vi "Sequencer Main - Copy.vi"() -> ()   [LabVIEW 2018] (continued)
                                }
                                frame True {
                                # "if(Retest-OFF & Cnt=0)"
                                n1515 = Decrement(x=w2562) -> (x-1=w2561:i32)
                                n1516 = global write "Global Variable.vi" "Retest Cnt"(w2561) -> ()
                                }
                                }
                                n1517 = global write "Global Variable.vi" "Retest ON"(TRUE ("Retest ON")) -> ()
                                }
                                }
                                }
                                frame True {
                                }
                              }
                            }
                          }
                        }
                        frame 42 {
                          # "BlueTooht Case\nEsp32 Reset"
                          # "Test ADB Bluetooth"
                          n1518 = Unbundle By Name(w2603) -> ("Parameters"=w2594:string, "Step Description"=w2591:string, "Test Values.Upper Limit"=w2598:dbl, "Test Values.Lower Limit"=w2597:dbl)  [unwired: 1 out]
                          n1519 = in-place {
                            in-place-border: w2594 -> [w2673]
                            in-place-border: [w2669] -> w2593
                            in-place-border: [w2668] -> w2592
                            # "Str \"fase\" exist"
                            n1520 = To Lower Case(string=w2673) -> (all lower case string=w2674:string)
                            n1521 = Match Pattern(string=w2674, regular expression="false") -> (after substring=w2671:string, offset past match=w2670:i32)  [unwired: 1 in, 2 out]
                            n1522 = Greater Or Equal To 0?(x=w2670) -> (x >= 0?=w2668:bool)
                            n1523 = case shown="True" w2668 {
                              tunnel: w2671 -> [_ w2677]
                              tunnel: [string[] [] w2676] -> w2669
                              frame False {
                                (unwired) ""
                              }
                              frame True {
                                n1524 = while {
                                shift-right: [w2681] -> _
                                shift-left: w2677 -> [w2682]
                                tunnel: [w2678] -> w2676 mode=indexing
                                stop <- w2680 stop-if-true
                                # "Get Array of Sub Parametrs"
                                n1525 = Match Pattern(string=w2682, regular expression=":") -> (before substring=w2678:string, after substring=w2681:string, offset past match=w2679:i32)  [unwired: 1 in, 1 out]
                                n1526 = Less Than 0?(x=w2679) -> (x < 0?=w2680:bool)
                                }
                              }
                            }
                          }
                          n1527 = property on="Msg Str" class="Str"("Value"=w2591) -> ()  [unwired: 2 in, 2 out]
                          n1528 = global read "Global Variable.vi" "COM Port BLE"() -> (w2588:refnum<visa-resource-name>)
                          n1529 = invoke on="Serial CMD Mon" class="Str" method="Reinit To Default"() -> (error out=w2587:errorcluster)  [unwired: 3 in, 2 out]
                          n1530 = property on="Tab Control Msg" class="TabCtl (strict)"("Value"=T4."Serial" ("Tab Control Msg")) -> (error out=w2601:errorcluster)  [unwired: 2 in, 1 out]
                          n1531 = flat-sequence {
                            tunnel: w2601 -> [w2611]
                            tunnel: w2598 -> [_]
                            tunnel: w2597 -> [_]
                            tunnel: w2594 -> [w2610]
                            tunnel: [w2612] -> w2596
                            tunnel: ["Reset ESP_32"] -> w2595
                            tunnel: w2591 -> [w2609]
                            tunnel: [w2604] -> w2590
                            tunnel: [w2608] -> w2589
                            tunnel: w2588 -> [w2607]
                            tunnel: w2587 -> [_]
                            tunnel: [w2632] -> w2599
                            tunnel: [w2638] -> w2602
                            tunnel: w2596 -> [w2638]
                            tunnel: w2595 -> [w2632]
                            tunnel: w2593 -> [w2637]
                            tunnel: w2592 -> [w2635]
                            tunnel: w2590 -> [w2631]
                            tunnel: w2589 -> [w2630]
                            frame #0 {
                              # "Step TEST Description"
                              # "Step TEST Result"
                              n1532 = in-place {
                                in-place-border: w2610 -> [w2619]
                                in-place-border: w2611 -> [_]
                                in-place-border: w2609 -> [w2617]
                                in-place-border: [w2616] -> w2604
                                in-place-border: [w2617] -> w2608
                                in-place-border: w2607 -> [w2618]
                                in-place-border: [w2615] -> w2605
                                # "ADB BLE Name"
                                n1533 = while {
                                shift-right: [w2627] -> _
                                shift-left: w2619 -> [w2628]
                                tunnel: [w2624] -> w2620 mode=indexing
                                stop <- w2626 stop-if-true
                                # "Get Array of Parametrs"
                                n1534 = Match Pattern(string=w2628, regular expression=">") -> (before substring=w2624:string, after substring=w2627:string, offset past match=w2625:i32)  [unwired: 1 in, 1 out]
                                n1535 = Less Than 0?(x=w2625) -> (x < 0?=w2626:bool)
                                }
                                n1536 = call "ADB-LMS_Esp32_Rst.vi"("COM BLE Esp32"=w2618) -> ("Stat"=w2615:bool, "CMD Monitor"=w2616:string)  [unwired: 9 in]
                                n1537 = Index Array(array=w2620, index #1=0 ("index"), index #2=1 ("index"), index #3=2 ("index")) -> ()  [unwired: 3 out]
                              }
                              n1538 = local write "Serial CMD Mon"(w2604) -> ()
                              n1539 = case shown="True" w2605 {
                                tunnel: [enum16{"Idle", "PASS", "FALSE"}."FALSE" ("Step Test Result") enum16{"Idle", "PASS", "FALSE"}."PASS" ("Step Test Result")] -> w2612
                                frame False {
                                }
                                frame True {
                                }
                              }
                            }
                            frame #1 {
                              # "Str \"fase\" Present"
                              n1540 = in-place {
                                in-place-border: w2630 -> [w2641]
                                in-place-border: w2631 -> [w2640]
                                in-place-border: w2632 -> [w2639]
                                n1541 = call "Log Add Msg.vi"("Result"=w2639, "Communication"=w2640, "Description"=w2641) -> ("Out Msg"=w2642:string)
                                n1542 = property on="LogMsg" class="Str"("Text.Scroll Position"=inf) -> ()  [unwired: 2 in, 2 out]
                                n1543 = invoke on="LogMsg" class="Str" method="Append String"("string"=w2642) -> ()  [unwired: 3 in, 4 out]
                              }
                              n1544 = in-place {
                                in-place-border: w2637 -> [w2667]
                                in-place-border: [w2661] -> w2634
                                in-place-border: [w2660] -> w2633
                                # "GoTo Test-nmb"
                                # "ReTest Cyckles"
                                n1545 = Index Array(array=w2667, index #1=0, index #2=1, index #3=2) -> (element #2=w2663:string, element #3=w2662:string)  [unwired: 1 out]
                                n1546 = Decimal String To Number(string=w2663) -> (number=w2661:i32)  [unwired: 2 in, 1 out]
                                n1547 = Decimal String To Number(string=w2662) -> (number=w2660:i32)  [unwired: 2 in, 1 out]
                              }
                              n1548 = local read "Debugging"() -> (w2636:bool)
                              n1549 = case shown="False" w2636 {
                                tunnel: w2635 -> [w2647 _]
                                tunnel: w2634 -> [w2645 _]
                                tunnel: w2633 -> [w2644 _]
                                frame False {
                                # "No Debug Mode"
                                n1550 = in-place {
                                in-place-border: [w2649] -> w2646
                                n1551 = global read "Global Variable.vi" "Retest Cnt"() -> (w2650:i16)
                                n1552 = Equal?(x=w2650, y=i16 0) -> (x = y?=w2649:bool)
                                }
                                n1553 = case shown="True" w2647 {
                                tunnel: w2646 -> [_ w2654]
                                tunnel: w2645 -> [_ w2652]
                                tunnel: w2644 -> [_ w2651]
                                frame False {
                                }
                                frame True {
                                # "String \"false\" Present"
                                n1554 = global write "Global Variable.vi" "Retest Step Nmb"(w2652) -> ()
                                n1555 = global write "Global Variable.vi" "Retest Nmb"(w2651) -> ()
                                n1556 = case shown="False" w2654 {
                                tunnel: w2651 -> [_ w2659]
                                frame False {
                                n1557 = global read "Global Variable.vi" "Retest Cnt"() -> (w2657:i16)
                                n1558 = Decrement(x=w2657) -> (x-1=w2656:i16)
                                n1559 = global write "Global Variable.vi" "Retest Cnt"(w2656) -> ()
                                n1560 = Wait (ms)(milliseconds to wait=u32 1000) -> ()  [unwired: 1 out]
                                }
                                frame True {
                                # "if(Retest-OFF & Cnt=0)"
                                n1561 = Decrement(x=w2659) -> (x-1=w2658:i32)
                                n1562 = global write "Global Variable.vi" "Retest Cnt"(w2658) -> ()
                                }
                                }
                                n1563 = global write "Global Variable.vi" "Retest ON"(TRUE ("Retest ON")) -> ()
                                }
                                }
                                }
                                frame True {
                                }
                              }
                            }
                          }
                        }
                        frame 43 {
                          w2700 = "------------------------" ("string")
                          w2699 = "\r\n"
                          # "Step TEST Result"
                          # "Step Result Msg"
                          # "Str with \"false\" goto parameters"
                          # "Str \"false\" Preset"
                          # "Cmd Case"
                          # "Cmd Case"
                          n1564 = Unbundle By Name(w2713) -> ("Parameters"=w2695:string, "Step Description"=w2684:string, "Test Values.Numeric Value"=w2689:dbl, "Test Values.Upper Limit"=w2688:dbl, "Test Values.Lower Limit"=w2687:dbl)
                          n1565 = in-place {
                            in-place-border: w2695 -> [w2745]
                            in-place-border: [w2744] -> w2694
                            in-place-border: [w2743] -> w2692
                            # "STr \"fase\" exist"
                            n1566 = To Lower Case(string=w2745) -> (all lower case string=w2746:string)
                            n1567 = Match Pattern(string=w2746, regular expression="false") -> (after substring=w2748:string, offset past match=w2749:i32)  [unwired: 1 in, 2 out]
                            n1568 = Greater Or Equal To 0?(x=w2749) -> (x >= 0?=w2743:bool)
                            n1569 = case shown="True" w2743 {
                              tunnel: w2748 -> [_ w2752]
                              tunnel: [string[] [] w2751] -> w2744
                              frame False {
                                (unwired) ""
                              }
                              frame True {
                                n1570 = while {
                                shift-right: [w2756] -> _
                                shift-left: w2752 -> [w2757]
                                tunnel: [w2753] -> w2751 mode=indexing
                                stop <- w2755 stop-if-true
                                # "Get Array of Sub Parametrs"
                                n1571 = Match Pattern(string=w2757, regular expression=":") -> (before substring=w2753:string, after substring=w2756:string, offset past match=w2754:i32)  [unwired: 1 in, 1 out]
                                n1572 = Less Than 0?(x=w2754) -> (x < 0?=w2755:bool)
                                }
                              }
                            }
                          }
                          n1573 = while {
                            shift-right: [w2762] -> _
                            shift-left: w2695 -> [w2763]
                            tunnel: [w2759] -> w2697 mode=indexing
                            stop <- w2761 stop-if-true
                            # "Get Array of Parametrs"
                            n1574 = Match Pattern(string=w2763, regular expression=">") -> (before substring=w2759:string, after substring=w2762:string, offset past match=w2760:i32)  [unwired: 1 in, 1 out]
                            n1575 = Less Than 0?(x=w2760) -> (x < 0?=w2761:bool)
                          }
                          n1576 = Concatenate Strings(w2684, w2699, w2700, w2700, w2700, w2699) -> (w2701:string)
                          n1577 = property on="Tab Control Msg" class="TabCtl (strict)"("Value"=T21."Serial" ("Tab Control Msg")) -> (error out=w2711:errorcluster)  [unwired: 2 in, 1 out]
                          n1578 = property on="Serial CMD Mon" class="Str"("Value"=w2701) -> ()  [unwired: 2 in, 2 out]
                          n1579 = Index Array(array=w2697, index=0) -> (element=w2709:string)
                          n1580 = Index Array(array=w2697, index=1) -> (element=w2707:string)
                          n1581 = Index Array(array=w2697, index=2) -> (element=w2704:string)
                          n1582 = Index Array(array=w2697, index=3) -> (element=w2702:string)
                          n1583 = Index Array(array=w2697, index=4) -> (element=w2696:string)
                          n1584 = case shown="\"getpid\"" w2709 {
                            tunnel: w2711 -> [_ _ _ _]
                            tunnel: [enum16{"Idle", "PASS", "FALSE"}."FALSE" ("Step Test Result") w2773 w2811 w2838] -> w2710
                            tunnel: w2707 -> [_ w2771 _ _]
                            tunnel: w2704 -> [_ _ _ _]
                            tunnel: w2702 -> [_ _ _ _]
                            tunnel: w2696 -> [_ _ _ _]
                            tunnel: ["" w2770 w2808 w2836] -> w2686
                            tunnel: w2689 -> [_ _ _ _]
                            tunnel: w2688 -> [_ _ _ _]
                            tunnel: w2687 -> [_ _ _ _]
                            tunnel: ["" w2769 w2810 w2835] -> w2685
                            frame "False", Default {
                              n1585 = One Button Dialog(message="!Sequencer File Err") -> ()  [unwired: 1 in, 1 out]
                            }
                            frame "open" {
                              # "Param"
                              # "Cmd"
                              n1586 = flat-sequence {
                                tunnel: [w2784] -> w2775
                                tunnel: [w2783] -> w2774
                                tunnel: [w2782] -> w2772
                                tunnel: w2775 -> [w2788]
                                tunnel: w2774 -> [w2790]
                                tunnel: [w2791] -> w2773
                                tunnel: w2772 -> [w2785]
                                tunnel: w2771 -> [w2789]
                                tunnel: [w2786] -> w2770
                                tunnel: [w2785] -> w2769
                                frame #0 {
                                n1587 = global read "Global Variable.vi" "COM Port FTDI RS232"() -> (w2781:refnum<visa-resource-name>)
                                n1588 = call "ADB-Serial_WrRd.vi"("Tx Deay"=u16 1, "Timeout(Sec)"=1.0, "PassString"="Chuck(1)", "Command"="open", "ComPort"=w2781) -> ("error out"=w2783:errorcluster, "PASS"=w2784:bool, "received"=w2782:string)  [unwired: 4 in]
                                n1589 = invoke on="Serial CMD Mon" class="Str" method="Append String"("string"=w2782) -> ()  [unwired: 3 in, 4 out]
                                n1590 = Wait (ms)(milliseconds to wait=u32 500) -> ()  [unwired: 1 out]
                                }
                                frame #1 {
                                n1591 = case shown="True" w2788 {
                                tunnel: w2785 -> [_ w2798]
                                tunnel: w2789 -> [_ w2804]
                                tunnel: [FALSE w2801] -> w2787
                                tunnel: ["!Firmware vertion not Right" ("line") w2797] -> w2786
                                frame False {
                                }
                                frame True {
                                n1592 = call <userlib>:"Multi-line String to Array__ogtk.vi"("string"=w2798) -> ("lines"=w2800:string[])
                                n1593 = To Lower Case(string=w2804) -> (all lower case string=w2803:string)
                                n1594 = To Lower Case(string=w2798) -> (all lower case string=w2805:string)
                                n1595 = Match Pattern(string=w2805, regular expression=w2803) -> (offset past match=w2802:i32)  [unwired: 1 in, 3 out]
                                n1596 = Index Array(array=w2800, index=2) -> (element=w2797:string)
                                n1597 = Greater Than 0?(x=w2802) -> (x > 0?=w2801:bool)
                                }
                                }
                                n1598 = global read "Global Variable.vi" "Array Errors"() -> (w2794:errorcluster[])
                                n1599 = Replace Array Subset(array=w2794, new element=w2790, index=3) -> (w2793:errorcluster[])
                                n1600 = global write "Global Variable.vi" "Array Errors"(w2793) -> ()
                                n1601 = case shown="True" w2787 {
                                tunnel: [enum16{"Idle", "PASS", "FALSE"}."FALSE" ("Step Test Result") enum16{"Idle", "PASS", "FALSE"}."PASS" ("Step Test Result")] -> w2791
                                frame False {
                                # "Step TEST Result"
                                }
                                frame True {
                                # "Step TEST Result"
                                }
                                }
                                }
                              }
                            }
                            frame "passwd" {
                              n1602 = flat-sequence {
                                tunnel: [w2822] -> w2813
                                tunnel: [w2821] -> w2812
                                tunnel: [w2820] -> w2809
                                tunnel: w2813 -> [w2825]
                                tunnel: w2812 -> [w2826]
                                tunnel: [w2827] -> w2811
                                tunnel: [w2824] -> w2810
                                tunnel: w2809 -> [w2824]
                                tunnel: [w2823] -> w2808
                                frame #0 {
                                n1603 = global read "Global Variable.vi" "COM Port FTDI RS232"() -> (w2819:refnum<visa-resource-name>)
                                n1604 = call "ADB-Serial_WrRd.vi"("Tx Deay"=u16 1, "Timeout(Sec)"=1.0, "PassString"="Chuck(3)", "Command"="passwd admin", "ComPort"=w2819) -> ("error out"=w2821:errorcluster, "PASS"=w2822:bool, "received"=w2820:string)  [unwired: 4 in]
                                n1605 = invoke on="Serial CMD Mon" class="Str" method="Append String"("string"=w2820) -> ()  [unwired: 3 in, 4 out]
                                n1606 = Wait (ms)(milliseconds to wait=u32 250) -> ()  [unwired: 1 out]
                                }
                                frame #1 {
                                n1607 = global read "Global Variable.vi" "Array Errors"() -> (w2830:errorcluster[])
                                n1608 = case shown="False" w2825 {
                                tunnel: [enum16{"Idle", "PASS", "FALSE"}."FALSE" ("Step Test Result") enum16{"Idle", "PASS", "FALSE"}."PASS" ("Step Test Result")] -> w2827
                                tunnel: ["Err" "Admin"] -> w2823
                                frame False {
                                # "Step TEST Result"
                                }
                                frame True {
                                # "Step TEST Result"
                                }
                                }
                                n1609 = Replace Array Subset(array=w2830, new element=w2826, index=3) -> (w2829:errorcluster[])
                                n1610 = global write "Global Variable.vi" "Array Errors"(w2829) -> ()
                                }
                              }
                            }
                            frame "getpid" {
                              # "Param"
                              # "Cmd"
                              n1611 = flat-sequence {
                                tunnel: [w2848] -> w2840
                                tunnel: [w2847] -> w2839
                                tunnel: [w2846] -> w2837
                                tunnel: [w2846] -> w2835
                                tunnel: w2840 -> [w2852]
                                tunnel: w2839 -> [w2855]
                                tunnel: [w2856] -> w2838
                                tunnel: [w2849] -> w2836
                                tunnel: w2837 -> [w2853]
                                frame #0 {
                                n1612 = global read "Global Variable.vi" "COM Port FTDI RS232"() -> (w2845:refnum<visa-resource-name>)
                                n1613 = global read "Global Variable.vi" "Wr PID"() -> (w2842:string)
                                n1614 = call "ADB-Serial_WrRd.vi"("Timeout(Sec)"=1.0, "PassString"=w2842, "Command"="getPID", "ComPort"=w2845) -> ("error out"=w2847:errorcluster, "PASS"=w2848:bool, "received"=w2846:string)  [unwired: 5 in]
                                n1615 = invoke on="Serial CMD Mon" class="Str" method="Append String"("string"=w2846) -> ()  [unwired: 3 in, 4 out]
                                n1616 = Wait (ms)(milliseconds to wait=u32 250) -> ()  [unwired: 1 out]
                                }
                                frame #1 {
                                n1617 = in-place {
                                in-place-border: w2855 -> [w2863]
                                in-place-border: [w2863] -> w2854
                                in-place-border: [w2864] -> w2850
                                in-place-border: w2853 -> [w2861]
                                n1618 = Match Pattern(string=w2861, regular expression="PID:" ("search string/char (-)")) -> (after substring=w2860:string)  [unwired: 1 in, 3 out]
                                n1619 = String Subset(string=w2860, offset (0)=1, length (rest)=13 ("length (rest)")) -> (substring=w2864:string)
                                n1620 = global write "Global Variable.vi" "Rd PID"(w2864) -> ()
                                }
                                n1621 = global read "Global Variable.vi" "Array Errors"() -> (w2859:errorcluster[])
                                n1622 = case shown="False" w2852 {
                                tunnel: [enum16{"Idle", "PASS", "FALSE"}."FALSE" ("Step Test Result") enum16{"Idle", "PASS", "FALSE"}."PASS" ("Step Test Result")] -> w2856
                                frame False {
                                # "Step TEST Result"
                                }
                                frame True {
                                # "Step TEST Result"
                                }
                                }
                                n1623 = Replace Array Subset(array=w2859, new element=w2854, index=3) -> (w2858:errorcluster[])
                                n1624 = global write "Global Variable.vi" "Array Errors"(w2858) -> ()
                                n1625 = Concatenate Strings("Read PID: " ("string"), w2850) -> (w2849:string)
                                }
                              }
                            }
                          }
                          n1626 = local read "Debugging"() -> (w2693:bool)
                          n1627 = in-place {
                            in-place-border: w2694 -> [w2737]
                            in-place-border: [w2736] -> w2690
                            in-place-border: [w2735] -> w2691
                            # "GoTo Test-nmb"
                            # "ReTest Cyckles"
                            n1628 = Index Array(array=w2737, index #1=0, index #2=1, index #3=2) -> (element #2=w2741:string, element #3=w2742:string)  [unwired: 1 out]
                            n1629 = Decimal String To Number(string=w2741) -> (number=w2736:i32)  [unwired: 2 in, 1 out]
                            n1630 = Decimal String To Number(string=w2742) -> (number=w2735:i32)  [unwired: 2 in, 1 out]
                          }
                          n1631 = case shown="False" w2693 {
                            tunnel: w2692 -> [w2722 _]
                            tunnel: w2690 -> [w2720 _]
                            tunnel: w2691 -> [w2719 _]
                            frame False {
                              # "No Debug Mode"
                              n1632 = in-place {
                                in-place-border: [w2724] -> w2721
                                n1633 = global read "Global Variable.vi" "Retest Cnt"() -> (w2725:i16)
                                n1634 = Equal?(x=w2725, y=i16 0) -> (x = y?=w2724:bool)
                              }
                              n1635 = case shown="True" w2722 {
                                tunnel: w2721 -> [_ w2729]
                                tunnel: w2720 -> [_ w2727]
                                tunnel: w2719 -> [_ w2726]
                                frame False {
                                }
                                frame True {
                                # "String \"false\" Present"
                                n1636 = global write "Global Variable.vi" "Retest Step Nmb"(w2727) -> ()
                                n1637 = global write "Global Variable.vi" "Retest Nmb"(w2726) -> ()
                                n1638 = case shown="False" w2729 {
                                tunnel: w2726 -> [_ w2734]
                                frame False {
                                n1639 = global read "Global Variable.vi" "Retest Cnt"() -> (w2732:i16)
                                n1640 = Decrement(x=w2732) -> (x-1=w2731:i16)
                                n1641 = global write "Global Variable.vi" "Retest Cnt"(w2731) -> ()
                                n1642 = Wait (ms)(milliseconds to wait=u32 1000) -> ()  [unwired: 1 out]
                                }
                                frame True {
                                # "if(Retest-OFF & Cnt=0)"
                                n1643 = Decrement(x=w2734) -> (x-1=w2733:i32)
                                n1644 = global write "Global Variable.vi" "Retest Cnt"(w2733) -> ()
                                }
                                }
                                n1645 = global write "Global Variable.vi" "Retest ON"(TRUE ("Retest ON")) -> ()
                                }
                              }
                            }
                            frame True {
                            }
                          }
                          n1646 = in-place {
                            in-place-border: w2684 -> [w2716]
                            in-place-border: w2685 -> [w2715]
                            in-place-border: w2686 -> [w2714]
                            n1647 = call "Log Add Msg.vi"("Result"=w2714, "Communication"=w2715, "Description"=w2716) -> ("Out Msg"=w2717:string)
                            n1648 = property on="LogMsg" class="Str"("Text.Scroll Position"=inf) -> ()  [unwired: 2 in, 2 out]
                            n1649 = invoke on="LogMsg" class="Str" method="Append String"("string"=w2717) -> ()  [unwired: 3 in, 4 out]
                          }
                        }
                        frame 45 {
                          # "Retest Cnt=0 ?"
                          # "RFID Case\nArduino"
                          # "Test ADB LMS RFID"
                          n1650 = Unbundle By Name(w2884) -> ("Test Values.Upper Limit"=w2878:dbl, "Test Values.Lower Limit"=w2879:dbl, "Parameters"=w2881:string)  [unwired: 2 out]
                          n1651 = property on="Tab Control Msg" class="TabCtl (strict)"("Value"=T4."Msg" ("Tab Control Msg")) -> (error out=w2882:errorcluster)  [unwired: 2 in, 1 out]
                          n1652 = in-place {
                            in-place-border: w2882 -> [_]
                            in-place-border: w2881 -> [w2925]
                            in-place-border: [w2917] -> w2880
                            in-place-border: w2879 -> [w2916]
                            in-place-border: w2878 -> [w2915]
                            in-place-border: [w2914] -> w2877
                            in-place-border: [w2912] -> w2876
                            # "COMPORT OPEN?"
                            n1653 = while {
                              shift-right: [w3227] -> _
                              shift-left: w2925 -> [w3228]
                              tunnel: [w3224] -> w2921 mode=indexing
                              stop <- w3226 stop-if-true
                              # "Get Array of Parametrs"
                              n1654 = Match Pattern(string=w3228, regular expression=">") -> (before substring=w3224:string, after substring=w3227:string, offset past match=w3225:i32)  [unwired: 1 in, 1 out]
                              n1655 = Less Than 0?(x=w3225) -> (x < 0?=w3226:bool)
                            }
                            n1656 = Index Array(array=w2921, index #1=0 ("index"), index #2=1 ("index"), index #3=2 ("index")) -> (element #1=w2913:string)  [unwired: 2 out]
                            n1657 = global read "Global Variable.vi" "COM Port RFID"() -> (w2920:refnum<visa-resource-name>)
                            n1658 = while {
                              shift-right: [w2929] -> _
                              shift-left: w2913 -> [w2930]
                              tunnel: [w2926] -> w2912 mode=indexing
                              stop <- w2928 stop-if-true
                              # "Get Array of Sub Parametrs"
                              n1659 = Match Pattern(string=w2930, regular expression=":") -> (before substring=w2926:string, after substring=w2929:string, offset past match=w2927:i32)  [unwired: 1 in, 1 out]
                              n1660 = Less Than 0?(x=w2927) -> (x < 0?=w2928:bool)
                            }
                            n1661 = Not Equal?(x=w2920, y="???") -> (x != y?=w2918:bool)
                            n1662 = case shown="True" w2918 {
                              tunnel: [FALSE w2942] -> w2917
                              tunnel: w2916 -> [_ w2944]
                              tunnel: w2915 -> [_ w2943]
                              tunnel: ["..." w2937] -> w2914
                              frame False {
                              }
                              frame True {
                                n1663 = flat-sequence {
                                tunnel: [w2968] -> w2940
                                tunnel: [w2964] -> w2934
                                tunnel: w2940 -> [w2995]
                                tunnel: [w2981] -> w2936
                                tunnel: [w2971] -> w2939
                                tunnel: [w2980] -> w2938
                                tunnel: w2934 -> [w2976]
                                frame #0 {
                                w2957 = "--------------------"
                                w2958 = "\r\n"
                                n1664 = case shown="True" FALSE {
                                frame False {
                                }
                                frame True {
                                n1665 = in-place {
                                # "Debug ONLY!"
                                n1666 = global write "Global Variable.vi" "Rd PID"("2119050000012") -> ()
                                }
                                }
                                }
                                n1667 = Concatenate Strings("Test ADB-LMS FRID", w2958, w2957, w2957, w2958, "Please WAIT  (Delay 10s)", w2958, w2957, w2957) -> (w2960:string)
                                n1668 = property on="Msg Str" class="Str"("Value"=w2960) -> ()  [unwired: 2 in, 2 out]
                                }
                                frame #1 {
                                n1669 = global read "Global Variable.vi" "COM Port RFID"() -> (w2963:refnum<visa-resource-name>)
                                n1670 = VISA Clear(VISA resource name=w2963) -> (VISA resource name out=w2967:refnum<visa-resource-name>, error out=w2966:errorcluster)  [unwired: 1 in]
                                n1671 = call "RFID Get ID.vi"("ComPort"=w2967) -> ("error out"=w2965:errorcluster, "received"=w2968:string)  [unwired: 9 in]
                                n1672 = invoke on="Msg Str" class="Str" method="Append String"("string"=w2968) -> ()  [unwired: 3 in, 4 out]
                                n1673 = Merge Errors(w2965, w2966) -> (w2964:errorcluster)
                                }
                                frame #2 {
                                w2990 = "\\[(.*)\\]" ("regular expression")
                                n1674 = call <userlib>:"Multi-line String to Array__ogtk.vi"("string"=w2995) -> ("lines"=w2994:string[])
                                n1675 = global read "Global Variable.vi" "Array Errors"() -> (w2979:errorcluster[])
                                n1676 = Index Array(array=w2994, index #1=1 ("index"), index #2=4 ("index")) -> (element #1=w2991:string, element #2=w2989:string)
                                n1677 = global read "Global Variable.vi" "Rd PID"() -> (w2974:string)
                                n1678 = xnode "Match Regular Expression"("input string"=w2989, "regular expression"=w2990) -> ("whole match"=w2985:string)  [unwired: 4 in, 4 out]
                                n1679 = xnode "Match Regular Expression"("input string"=w2991, "regular expression"=w2990) -> ("whole match"=w2987:string)  [unwired: 4 in, 4 out]
                                n1680 = Replace Array Subset(array=w2979, new element=w2976, index=7) -> (w2978:errorcluster[])
                                n1681 = global write "Global Variable.vi" "Array Errors"(w2978) -> ()
                                n1682 = String Subset(string=w2987, offset (0)=1, length (rest)=3 ("offset (0)")) -> (substring=w2975:string)
                                n1683 = String Subset(string=w2985, offset (0)=8, length (rest)=13 ("length (rest)")) -> (substring=w2971:string)
                                n1684 = Decimal String To Number(string=w2975) -> (number=w2980:i32)  [unwired: 2 in, 1 out]
                                n1685 = Concatenate Strings("rssi: ", w2975, "db Rd-PID: <", w2974, ">", "\r\n", "RFID-PID: " ("string"), w2971) -> (w2981:string)
                                }
                                }
                                n1686 = in-place {
                                in-place-border: [w2954] -> w2935
                                in-place-border: w2939 -> [w2953]
                                n1687 = global read "Global Variable.vi" "Rd PID"() -> (w2955:string)
                                n1688 = Equal?(x=w2955, y=w2953) -> (x = y?=w2954:bool)
                                n1689 = global write "Global Variable.vi" "Rd PID RFID"(w2953) -> ()
                                }
                                n1690 = case shown="False" w2935 {
                                tunnel: [w2947 w2948] -> w2937
                                tunnel: w2936 -> [w2946 w2948]
                                frame False {
                                n1691 = Concatenate Strings(w2946, " (False)" ("string")) -> (w2947:string)
                                }
                                frame True {
                                }
                                }
                                n1692 = in-place {
                                in-place-border: w2938 -> [w2950]
                                in-place-border: w2943 -> [w2952]
                                in-place-border: w2944 -> [w2951]
                                in-place-border: [w2949] -> w2941
                                n1693 = In Range and Coerce(upper limit=w2952, x=w2950, lower limit=w2951) -> (In Range?=w2949:bool)  [unwired: 1 out]
                                }
                                n1694 = And(x=w2941, y=w2935) -> (x .and. y?=w2942:bool)
                              }
                            }
                          }
                          n1695 = local read "Debugging"() -> (w2872:bool)
                          n1696 = global read "Global Variable.vi" "Retest Cnt"() -> (w2874:i16)
                          n1697 = in-place {
                            in-place-border: w2876 -> [w2905]
                            in-place-border: [w2904] -> w2875
                            in-place-border: [w2903] -> w2870
                            in-place-border: [w2902] -> w2869
                            # "GoTo Test-nmb"
                            # "ReTest Cyckles"
                            n1698 = Index Array(array=w2905, index #1=0 ("index"), index #2=1 ("index"), index #3=2 ("index")) -> (element #1=w2908:string, element #2=w2907:string, element #3=w2906:string)
                            n1699 = Decimal String To Number(string=w2906) -> (number=w2903:i32)  [unwired: 2 in, 1 out]
                            n1700 = Decimal String To Number(string=w2907) -> (number=w2902:i32)  [unwired: 2 in, 1 out]
                            n1701 = To Upper Case(1:w2908) -> (0:w2904:string)
                          }
                          n1702 = case shown="True" w2880 {
                            tunnel: [enum16{"Idle", "PASS", "FALSE"}."FALSE" ("Step Test Result") enum16{"Idle", "PASS", "FALSE"}."PASS" ("Step Test Result")] -> w2885
                            frame False {
                            }
                            frame True {
                            }
                          }
                          n1703 = Equal?(x=w2874, y=i16 0) -> (x = y?=w2871:bool)
                          n1704 = case shown="False" w2872 {
                            tunnel: w2875 -> [w2889 _]
                            tunnel: w2871 -> [w2886 _]
                            tunnel: w2870 -> [w2888 _]
                            tunnel: w2869 -> [w2887 _]
                            frame False {
                              n1705 = case shown="\"FALSE\"" w2889 {
                                tunnel: w2886 -> [_ w2890]
                                tunnel: w2888 -> [_ w2892]
                                tunnel: w2887 -> [_ w2891]
                                frame "Idle", Default {
                                }
                                frame "FALSE" {
                                n1706 = case shown="False" w2890 {
                                tunnel: w2892 -> [_ w2899]
                                tunnel: w2891 -> [w2894 w2901]
                                frame False {
                                n1707 = global read "Global Variable.vi" "Retest Cnt"() -> (w2897:i16)
                                n1708 = global write "Global Variable.vi" "Retest Step Nmb"(w2894) -> ()
                                n1709 = global write "Global Variable.vi" "Retest ON"(TRUE ("Retest ON")) -> ()
                                n1710 = Decrement(x=w2897) -> (x-1=w2896:i16)
                                n1711 = global write "Global Variable.vi" "Retest Cnt"(w2896) -> ()
                                n1712 = Wait (ms)(milliseconds to wait=u32 1000) -> ()  [unwired: 1 out]
                                }
                                frame True {
                                # "if(Retest-OFF & Cnt=0)"
                                n1713 = Decrement(x=w2899) -> (x-1=w2898:i32)
                                n1714 = global write "Global Variable.vi" "Retest Step Nmb"(w2901) -> ()
                                n1715 = global write "Global Variable.vi" "Retest ON"(TRUE ("Retest ON")) -> ()
                                n1716 = global write "Global Variable.vi" "Retest Cnt"(w2898) -> ()
                                }
                                }
                                }
                              }
                            }
                            frame True {
                            }
                          }
                        }
                        frame 46 {
                          # "GoTo Test-nmb"
                          # "ReTest Cyckles"
                          # "RFID Case\nFTDI"
                          # "Test ADB LMS RFID"
                          n1717 = Unbundle By Name(w3248) -> ("Test Values.Upper Limit"=w3242:dbl, "Test Values.Lower Limit"=w3243:dbl, "Parameters"=w3245:string, "Step Description"=w3234:string)  [unwired: 1 out]
                          n1718 = property on="Tab Control Msg" class="TabCtl (strict)"("Value"=T4."Msg" ("Tab Control Msg")) -> (error out=w3246:errorcluster)  [unwired: 2 in, 1 out]
                          n1719 = in-place {
                            in-place-border: w3246 -> [_]
                            in-place-border: w3245 -> [w3294]
                            in-place-border: [w3288] -> w3244
                            in-place-border: w3243 -> [w3287]
                            in-place-border: w3242 -> [w3286]
                            in-place-border: [w3285] -> w3235
                            in-place-border: [w3283] -> w3241
                            in-place-border: w3234 -> [w3282]
                            in-place-border: [w3282] -> w3233
                            in-place-border: [w3281] -> w3232
                            n1720 = while {
                              shift-right: [w3478] -> _
                              shift-left: w3294 -> [w3479]
                              tunnel: [w3475] -> w3290 mode=indexing
                              stop <- w3477 stop-if-true
                              # "Get Array of Parametrs"
                              n1721 = Match Pattern(string=w3479, regular expression=">") -> (before substring=w3475:string, after substring=w3478:string, offset past match=w3476:i32)  [unwired: 1 in, 1 out]
                              n1722 = Less Than 0?(x=w3476) -> (x < 0?=w3477:bool)
                            }
                            n1723 = Index Array(array=w3290, index #1=0 ("index"), index #2=1 ("index"), index #3=2 ("index")) -> (element #1=w3284:string)  [unwired: 2 out]
                            n1724 = in-place {
                              in-place-border: [w3295] -> w3289
                              # "COMPORT OPEN?"
                              n1725 = global read "Global Variable.vi" "COM Port RFID"() -> (w3297:refnum<visa-resource-name>)
                              n1726 = Not Equal?(x=w3297, y="???") -> (x != y?=w3295:bool)
                            }
                            n1727 = while {
                              shift-right: [w3301] -> _
                              shift-left: w3284 -> [w3302]
                              tunnel: [w3298] -> w3283 mode=indexing
                              stop <- w3300 stop-if-true
                              # "Get Array of Sub Parametrs"
                              n1728 = Match Pattern(string=w3302, regular expression=":") -> (before substring=w3298:string, after substring=w3301:string, offset past match=w3299:i32)  [unwired: 1 in, 1 out]
                              n1729 = Less Or Equal To 0?(x=w3299) -> (x <= 0?=w3300:bool)
                            }
                            n1730 = case shown="True" w3289 {
                              tunnel: [FALSE w3317] -> w3288
                              tunnel: w3287 -> [_ w3319]
                              tunnel: w3286 -> [_ w3318]
                              tunnel: [w3304 w3307] -> w3285
                              tunnel: [w3304 w3306] -> w3281
                              frame False {
                                w3304 = "..."
                              }
                              frame True {
                                n1731 = flat-sequence {
                                tunnel: [w3337] -> w3315
                                tunnel: [w3339] -> w3310
                                tunnel: [w3338] -> w3309
                                tunnel: [w3337] -> w3308
                                tunnel: w3315 -> [w3354]
                                tunnel: [w3359] -> w3312
                                tunnel: [w3345] -> w3314
                                tunnel: [w3353] -> w3313
                                tunnel: w3310 -> [w3355]
                                tunnel: w3309 -> [w3353]
                                tunnel: w3308 -> [w3344]
                                tunnel: [w3344] -> w3306
                                frame #0 {
                                w3332 = "--------------------"
                                w3333 = "\r\n"
                                n1732 = case shown="True" FALSE {
                                frame False {
                                }
                                frame True {
                                n1733 = in-place {
                                # "Debug ONLY!"
                                n1734 = global write "Global Variable.vi" "Rd PID"("2205040012345") -> ()
                                }
                                }
                                }
                                n1735 = Concatenate Strings("Test ADB-LMS FRID", w3333, w3332, w3332, w3333) -> (w3334:string)
                                n1736 = property on="Msg Str" class="Str"("Value"=w3334) -> ()  [unwired: 2 in, 2 out]
                                }
                                frame #1 {
                                n1737 = global read "Global Variable.vi" "COM Port RFID"() -> (w3343:refnum<visa-resource-name>)
                                n1738 = VISA Clear(VISA resource name=w3343) -> (VISA resource name out=w3342:refnum<visa-resource-name>, error out=w3341:errorcluster)  [unwired: 1 in]
                                n1739 = call "RFID_FTDI_Get-ID.vi"("error in"=w3341, "Delay"=u16 1200, "COM RFID"=w3342) -> ("error out"=w3339:errorcluster, "RSSI"=w3338:i32, "Str EPC"=w3337:string)  [unwired: 5 in, 1 out]
                                n1740 = invoke on="Msg Str" class="Str" method="Append String"("string"=w3337) -> ()  [unwired: 3 in, 4 out]
                                }
                                frame #2 {
                                # "RFID PID"
                                n1741 = global read "Global Variable.vi" "Array Errors"() -> (w3358:errorcluster[])
                                n1742 = xnode "Match Regular Expression"("input string"=w3354, "regular expression"="\\[(.*)\\]") -> ("whole match"=w3352:string)  [unwired: 4 in, 4 out]
                                n1743 = Number To Decimal String(number=w3353) -> (decimal integer string=w3349:string)  [unwired: 1 in]
                                n1744 = String Subset(string=w3352, offset (0)=8, length (rest)=13 ("offset (0)")) -> (substring=w3345:string)
                                n1745 = Replace Array Subset(array=w3358, new element=w3355, index=7) -> (w3357:errorcluster[])
                                n1746 = global write "Global Variable.vi" "Array Errors"(w3357) -> ()
                                n1747 = Concatenate Strings(w3349, " (db) ", "\r\n", "                   RFID-PID: " ("string"), w3345) -> (w3359:string)
                                }
                                }
                                n1748 = in-place {
                                in-place-border: [w3330] -> w3311
                                in-place-border: w3314 -> [w3329]
                                n1749 = global read "Global Variable.vi" "Rd PID"() -> (w3328:string)
                                n1750 = global write "Global Variable.vi" "Rd PID RFID"(w3329) -> ()
                                n1751 = Equal?(x=w3328, y=w3329) -> (x = y?=w3330:bool)
                                }
                                n1752 = case shown="True" w3311 {
                                tunnel: [w3322 w3323] -> w3307
                                tunnel: w3312 -> [w3321 w3323]
                                frame False {
                                n1753 = Concatenate Strings(w3321, " (False)" ("string")) -> (w3322:string)
                                }
                                frame True {
                                }
                                }
                                n1754 = in-place {
                                in-place-border: w3313 -> [w3325]
                                in-place-border: w3318 -> [w3327]
                                in-place-border: w3319 -> [w3326]
                                in-place-border: [w3324] -> w3316
                                n1755 = In Range and Coerce(upper limit=w3327, x=w3325, lower limit=w3326) -> (In Range?=w3324:bool)  [unwired: 1 out]
                                }
                                n1756 = And(x=w3316, y=w3311) -> (x .and. y?=w3317:bool)
                              }
                            }
                          }
                          n1757 = local read "Debugging"() -> (w3239:bool)
                          n1758 = in-place {
                            in-place-border: w3241 -> [w3274]
                            in-place-border: [w3273] -> w3240
                            in-place-border: [w3272] -> w3236
                            in-place-border: [w3271] -> w3237
                            n1759 = Index Array(array=w3274, index #1=0 ("index"), index #2=1 ("index"), index #3=2 ("index")) -> (element #1=w3277:string, element #2=w3276:string, element #3=w3275:string)
                            n1760 = Decimal String To Number(string=w3275) -> (number=w3272:i32)  [unwired: 2 in, 1 out]
                            n1761 = Decimal String To Number(string=w3276) -> (number=w3271:i32)  [unwired: 2 in, 1 out]
                            n1762 = To Upper Case(1:w3277) -> (0:w3273:string)
                          }
                          n1763 = in-place {
                            in-place-border: [w3256] -> w3238
                            n1764 = global read "Global Variable.vi" "Retest Cnt"() -> (w3257:i16)
                            n1765 = Equal?(x=w3257, y=i16 0) -> (x = y?=w3256:bool)
                          }
                          n1766 = case shown="False" w3239 {
                            tunnel: w3240 -> [w3261 _]
                            tunnel: w3238 -> [w3258 _]
                            tunnel: w3236 -> [w3260 _]
                            tunnel: w3237 -> [w3259 _]
                            frame False {
                              # "Debug ?"
                              n1767 = case shown="\"FALSE\"" w3261 {
                                tunnel: w3258 -> [_ w3265]
                                tunnel: w3260 -> [_ w3262]
                                tunnel: w3259 -> [_ w3263]
                                frame "Idle", Default {
                                }
                                frame "FALSE" {
                                # "If \"false\" para exixst?"
                                n1768 = global write "Global Variable.vi" "Retest Step Nmb"(w3263) -> ()
                                n1769 = global write "Global Variable.vi" "Retest Nmb"(w3262) -> ()
                                n1770 = case shown="True" w3265 {
                                tunnel: w3262 -> [_ w3270]
                                frame False {
                                # "Else"
                                n1771 = global read "Global Variable.vi" "Retest Cnt"() -> (w3268:i16)
                                n1772 = Decrement(x=w3268) -> (x-1=w3267:i16)
                                n1773 = global write "Global Variable.vi" "Retest Cnt"(w3267) -> ()
                                n1774 = Wait (ms)(milliseconds to wait=u32 1000) -> ()  [unwired: 1 out]
                                }
                                frame True {
                                # "if(Retest-OFF & Cnt=0)"
                                n1775 = Decrement(x=w3270) -> (x-1=w3269:i32)
                                n1776 = global write "Global Variable.vi" "Retest Cnt"(w3269) -> ()
                                }
                                }
                                n1777 = global write "Global Variable.vi" "Retest ON"(TRUE ("Retest ON")) -> ()
                                }
                              }
                            }
                            frame True {
                            }
                          }
                          n1778 = in-place {
                            in-place-border: w3233 -> [w3252]
                            in-place-border: w3232 -> [w3251]
                            in-place-border: w3235 -> [w3250]
                            n1779 = call "Log Add Msg.vi"("Result"=w3250, "Communication"=w3251, "Description"=w3252) -> ("Out Msg"=w3253:string)
                            n1780 = property on="LogMsg" class="Str"("Text.Scroll Position"=inf) -> ()  [unwired: 2 in, 2 out]
                            n1781 = invoke on="LogMsg" class="Str" method="Append String"("string"=w3253) -> ()  [unwired: 3 in, 4 out]
                          }
                          n1782 = case shown="False" w3244 {
                            tunnel: [enum16{"Idle", "PASS", "FALSE"}."FALSE" ("Step Test Result") enum16{"Idle", "PASS", "FALSE"}."PASS" ("Step Test Result")] -> w3249
                            frame False {
                            }
                            frame True {
